vi "Run Bfr Rx - PingPong - Change Flush Add.vi"(4 "Data Size in":u64, 6 "Change Active":bool, 7 "Buffer_A":u64 format="%016x", 8 "error in (no error)":errorcluster, 10 "Data in":u8[](array[numeric]), 11 "Ping Pong Buffer in":T1 {"Active Buffer Ref" format="%016x"}) -> (0 "error out":errorcluster, 3 "Ping Pong Buffer out":T1 {"Active Buffer Ref" format="%016x"})   [LabVIEW 2019, in "UDP-Custom-Device Engine.lvlib"]
uses:
  UDP-Custom-Device Engine.lvlib
  Types/Engine - Buffered Rx Ping Pong Buffer.ctl
  Types/Engine - Buffered Rx Active Buffer.ctl
  <vilib>/NI VeriStand/VeriStand Data/Pointer Operations/Pointer.Write.vi
  <vilib>/NI VeriStand/VeriStand Data/Pointer Operations/Pointer.Write (1D U8).vi
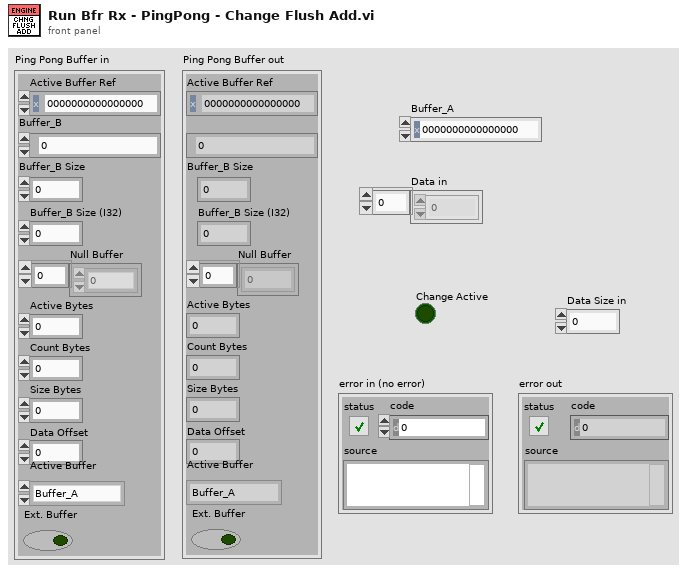
[diagram p1: front panel]
types:
  T1 = typedef "UDP-Custom-Device Engine.lvlib/Engine - Buffered Rx Ping Pong Buffer.ctl" = cluster{"Active Buffer Ref":u64, "Buffer_B":u64, "Buffer_B Size":u64, "Buffer_B Size (I32)":i32, "Null Buffer":u8[], "Active Bytes":u64, "Count Bytes":u64, "Size Bytes":u64, "Data Offset":u64, "Active Buffer":T2, "Ext. Buffer":bool}
  T2 = typedef "UDP-Custom-Device Engine.lvlib/Engine - Buffered Rx Active Buffer.ctl" = enum16{"Buffer_A", "Buffer_B"}
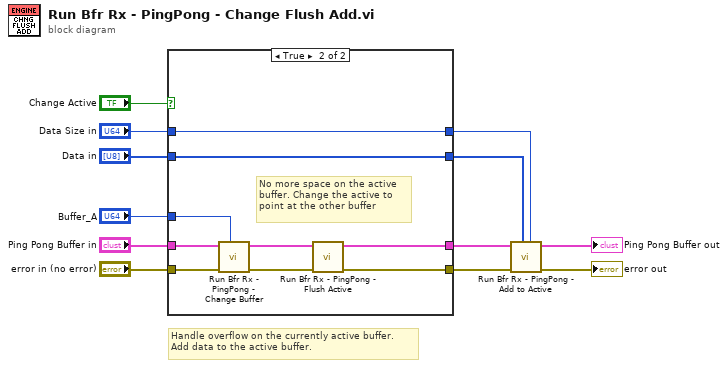
[diagram p0: block diagram]
diagram:
  # "Handle overflow on the currently active buffer.\nAdd data to the active buffer."
  n1 = case shown="True" "Change Active" {
    tunnel: "Ping Pong Buffer in" -> [w14 w22]
    tunnel: "error in (no error)" -> [w15 w23]
    tunnel: "Buffer_A" -> [_ w21]
    tunnel: "Data Size in" -> [w13 w24]
    tunnel: "Data in" -> [w16 w25]
    tunnel: [w16 w25] -> w6
    tunnel: [w15 w17] -> w3
    tunnel: [w14 w19] -> w1
    tunnel: [w13 w24] -> w5
    frame False {
      # "There is still space to write\ndata in the active buffer. Skip\nchanging the active buffer and\nadd the new data."
    }
    frame True {
      # "No more space on the active\nbuffer. Change the active to\npoint at the other buffer"
      n2 = call "Run Bfr Rx - PingPong - Change Buffer.vi"("Buffer_A"=w21, "error in (no error)"=w23, "Ping Pong Buffer in"=w22) -> ("error out"=w18:errorcluster, "Ping Pong Buffer out"=w20:T1)  [unwired: 7 in]
      n3 = call "Run Bfr Rx - PingPong - Flush Active.vi"("error in (no error)"=w18, "Ping Pong Buffer in"=w20) -> ("error out"=w17:errorcluster, "Ping Pong Buffer out"=w19:T1)  [unwired: 8 in]
    }
  }
  n4 = call "Run Bfr Rx - PingPong - Add to Active.vi"("Data Size in"=w5, "Data in"=w6, "error in (no error)"=w3, "Ping Pong Buffer in"=w1) -> ("error out"=→"error out":errorcluster, "Ping Pong Buffer out"=→"Ping Pong Buffer out":T1)  [unwired: 6 in]
